vi "After File Logging.vi"(4 "Delimiter":string=",", 6 "List Folder Pattern":string="*.csv", 8 "Error In":errorcluster, 11 "Test Log Folder":path=path "") -> (0 "Error Out":errorcluster, 3 "Records":string[][](array[string]))   [LabVIEW 2018, in "Tests.lvlib"]
uses:
  Tests.lvlib
  src/Toolkit/Support/Control State.vi
  <vilib>/Utility/file.llb/Read Delimited Spreadsheet (string).vi
  src/Toolkit/Toolkit.lvlib
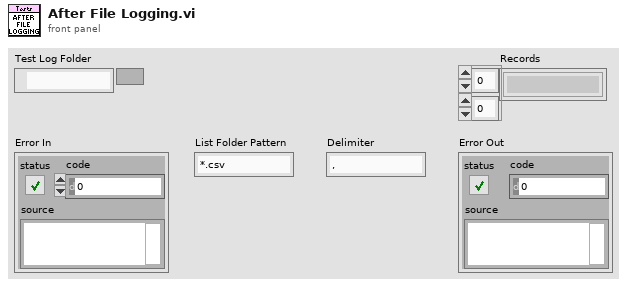
[diagram p1: front panel]
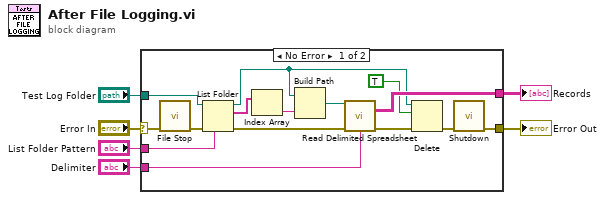
[diagram p0: block diagram]
diagram:
  n1 = case shown="No Error" "Error In" {
    selector: "Error In" -> [w10 w22]
    tunnel: "Delimiter" -> [w21 _]
    tunnel: [w20 _] -> w5
    tunnel: [w7 w22] -> w4
    tunnel: "List Folder Pattern" -> [w12 _]
    tunnel: "Test Log Folder" -> [w11 _]
    frame No Error {
      n2 = call "File Stop.vi"("Error In"=w10) -> ("Error Out"=w9:errorcluster)  [unwired: 10 in]
      n3 = List Folder(path=w11, pattern=w12, error in=w9) -> (path out=w15:path, filenames=w14:string[], error out=w18:errorcluster)  [unwired: 1 in, 1 out]
      n4 = Index Array(array=w14) -> (element=w16:string)  [unwired: 1 in]
      n5 = Build Path(base path=w15, name or relative path=w16) -> (appended path=w17:path)
      n6 = call-poly <vilib>:"Read Delimited Spreadsheet.vi"("file path (dialog if empty)"=w17, "error in (no error)"=w18, "delimiter (\\t)"=w21) -> ("all rows"=w20:string[][], "error out"=w19:errorcluster)  [unwired: 7 in, 4 out]
      n7 = Delete(path (use dialog)=w15, entire hierarchy (F)=TRUE, error in=w19) -> (error out=w8:errorcluster)  [unwired: 2 in, 2 out]
      n8 = call "Shutdown.vi"("Error In"=w8) -> ("Error Out"=w7:errorcluster)  [unwired: 10 in]
    }
    frame Error {
    }
  }
  "Records" <- w5
  "Error Out" <- w4
